vi "Load.vi"(0 "iUser Configuration Manager":refnum<class "iUser Configuration Manager.lvclass">, 5 "Username":string, 7 "Password":string, 9 "Path":path, 11 "error in (no error)":errorcluster, 12 "Persistence":refnum<class "IPersist.lvclass">) -> (4 "iUser Configuration Manager.lvclass":refnum<class "iUser Configuration Manager.lvclass">, 6 "Verified":bool, 8 "Verification Message":string, 15 "error out":errorcluster)   [LabVIEW 2017, in "User Configuration Manager.lvlib" / "iUser Configuration Manager.lvclass"]
doc: "Loads the User Configuration Manager from disk and logs in using the credentials specified. A user with the credentials specified must exist in the User Configuration Manager."
uses:
  iUser Configuration Manager.lvclass
  <vilib>/gpm_packages/@cs/persistence/source/IPersist/IPersist.lvclass
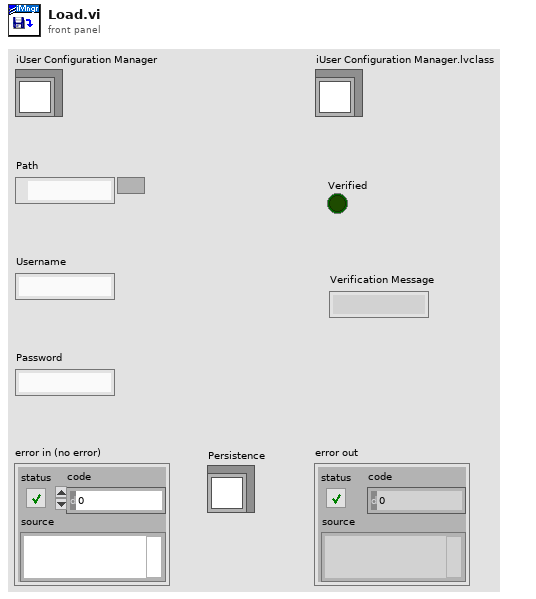
[diagram p1: front panel]
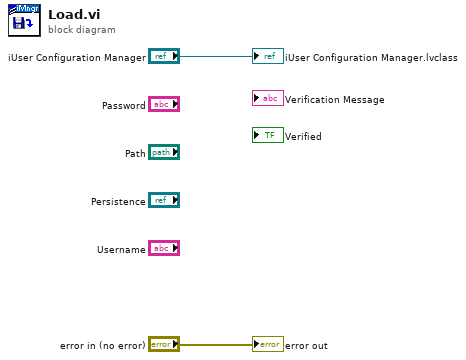
[diagram p0: block diagram]
diagram:
  "iUser Configuration Manager.lvclass" <- "iUser Configuration Manager"
  "error out" <- "error in (no error)"
